vi "Write Value as Variant.vi"(8 "error in (no error)":errorcluster, 9 "Variant":variant, 10 "Tag":string, 11 "Var Bus in":refnum<class "Multi_Bus.lvclass">) -> (0 "error out":errorcluster, 3 "Var Bus out":refnum<class "Multi_Bus.lvclass">)   [LabVIEW 2021, in "Multi_Bus.lvclass"]
uses:
  Multi_Bus.lvclass
  <vilib>/TSA/Abstract Data Classes/Abs_Types/Value/Abs_Value.lvclass
  Multi_Bus.lvclass/Multi_Bus.ctl
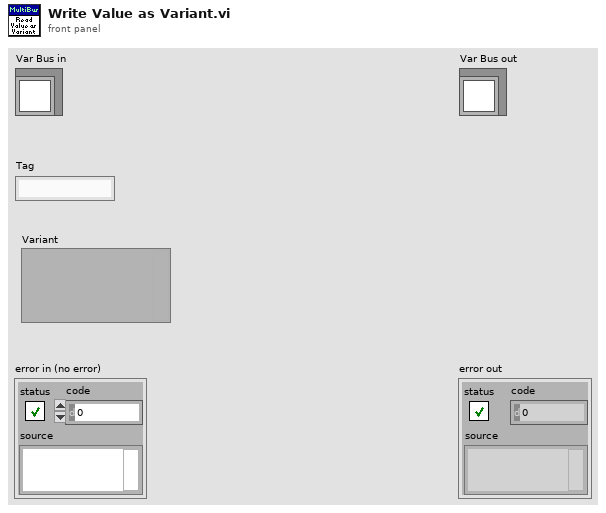
[diagram p1: front panel]
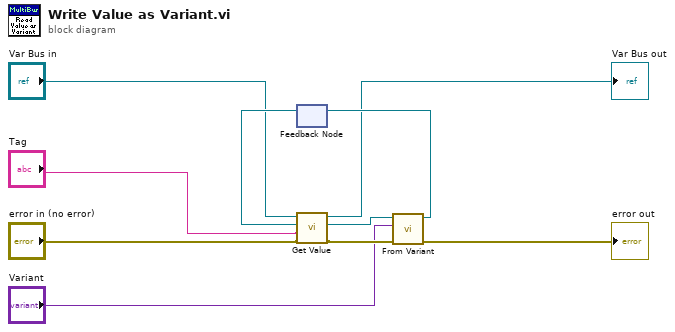
[diagram p0: block diagram]
diagram:
  n1 = feedback #1() -> (w4:refnum<class "Abs_Value.lvclass">)  [unwired: 1 in]
  n2 = call-dynamic "Get Value.vi"("error in (no error)"="error in (no error)", "Tag"="Tag", "Value Type"=w4, "Var Bus in"="Var Bus in") -> ("error out"=w8:errorcluster, "Value Out"=w7:refnum<class "Abs_Value.lvclass">, "Var Bus out"=→"Var Bus out":refnum<class "Multi_Bus.lvclass">)  [unwired: 5 in]
  n3 = call-dynamic "From Variant.vi"("error in (no error)"=w8, "Variant"="Variant", "Abs_Value in"=w7) -> ("error out"=→"error out":errorcluster, "Abs_Value out"=w9:refnum<class "Abs_Value.lvclass">)  [unwired: 7 in]
  n4 = feedback-in #1(w9) -> ()
